vi "subDFD_Close VIs.vi"(8 "error in (no error)":errorcluster, 11 "all VIs refs":refnum<vi>[](array[refnum])) -> (0 "error out":errorcluster)   [LabVIEW 2023]
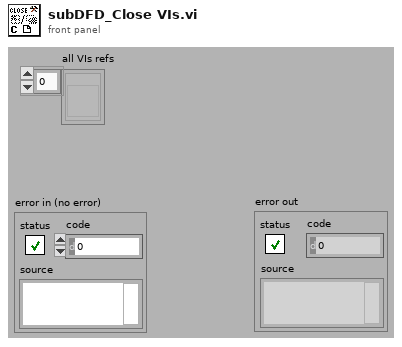
[diagram p1: front panel]
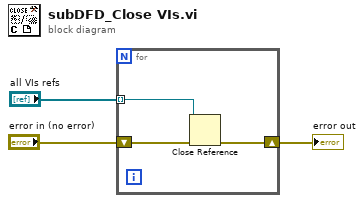
[diagram p0: block diagram]
diagram:
  n1 = for {
    shift-right: [w5] -> w2
    shift-left: "error in (no error)" -> [w6]
    tunnel: "all VIs refs" -> [w4] mode=indexing
    n2 = Close Reference(reference=w4, error in (no error)=w6) -> (error out=w5:errorcluster)
  }
  "error out" <- w2
